vi "Device.compactDAQ.Find.vi"(8 "error in (no error)":errorcluster) -> (0 "error out":errorcluster, 3 "compactDAQ":tag)   [LabVIEW 2018]
uses:
  <resource>/objmgr/daqmx.rc
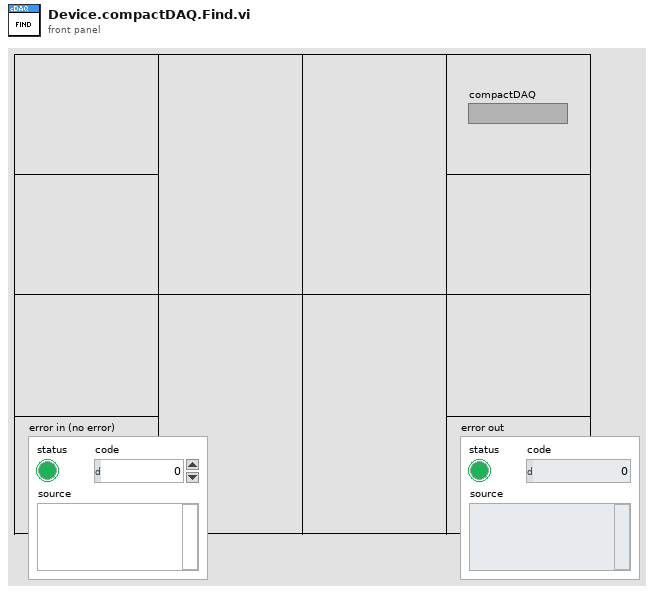
[diagram p1: front panel]
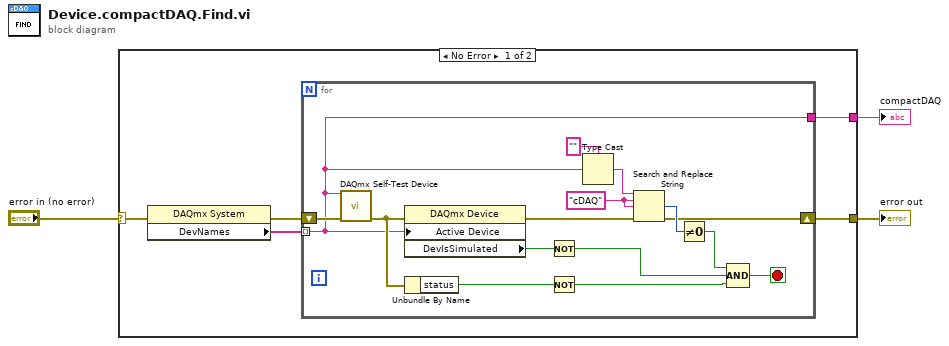
[diagram p0: block diagram]
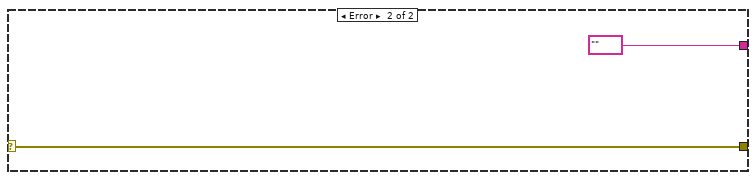
[diagram p2: hidden frame]
diagram:
  n1 = case shown="No Error" "error in (no error)" {
    selector: "error in (no error)" -> [w8 w25]
    tunnel: [w6 w25] -> w3
    tunnel: [w4 tag ""] -> w1
    frame No Error {
      n2 = property class="DAQmx System"(error in=w8) -> (error out=w7:errorcluster, "DevNames"=w5:tag[])  [unwired: 1 in, 1 out]
      n3 = for {
        shift-right: [w14] -> w6
        shift-left: w7 -> [w19]
        tunnel: w5 -> [w9] mode=indexing
        tunnel: [w9] -> w4
        stop <- w13 stop-if-true
        w21 = "cDAQ"
        n4 = call <vilib>:"DAQmx Self-Test Device.vi"("device in"=w9, "error in"=w19) -> ("error out"=w18:errorcluster)  [unwired: 13 in]
        n5 = property class="DAQmx Device"(error in=w18, "Active Device"=w9) -> (error out=w15:errorcluster, "DevIsSimulated"=w16:bool)  [unwired: 1 in, 1 out]
        n6 = Unbundle By Name(w18) -> ("status"=w17:bool)
        n7 = Not(x=w16) -> (.not. x?=w11:bool)
        n8 = Not(x=w17) -> (.not. x?=w12:bool)
        n9 = Type Cast(type="", x=w9) -> (*(type *) &x=w23:string)
        n10 = Search and Replace String(input string=w23, search string=w21, replace string=w21, error in=w15) -> (number of replacements=w20:i32, error out=w14:errorcluster)  [unwired: 4 in, 2 out]
        n11 = Not Equal To 0?(x=w20) -> (x != 0?=w10:bool)
        n12 = Compound Arithmetic op=AND(w10, w11, w12) -> (w13:bool)
      }
    }
    frame Error {
    }
  }
  "error out" <- w3
  "compactDAQ" <- w1
